vi "GetProgress.vi"(8 "error in (no error)":errorcluster, 11 "Progress in":refnum<class "Progress.lvclass">) -> (0 "error out":errorcluster, 2 "Progress":u64, 3 "Progress out":refnum<class "Progress.lvclass">)   [LabVIEW 2021, in "Progress.lvlib" / "Progress.lvclass"]
uses:
  Progress.lvclass
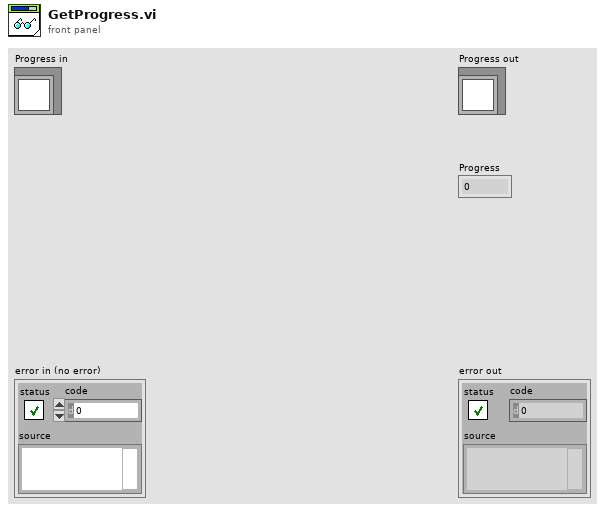
[diagram p1: front panel]
types:
  T1 = typedef "Progress.lvlib/Progress.lvclass/Data.ctl" = cluster{"SlideRefnum":refnum<vi>, "ProgressValue":u64, "NbElement":u64, "Caption":string, "UINotifier":refnum<notifier>, "StopUI":refnum<user-event>}
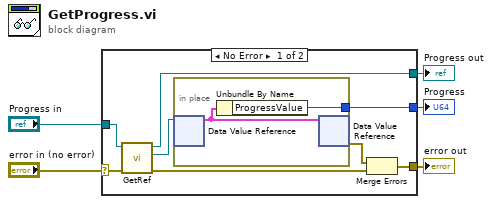
[diagram p0: block diagram]
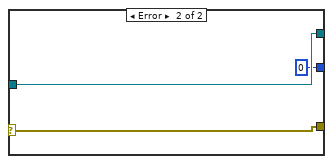
[diagram p2: hidden frame]
diagram:
  n1 = case shown="No Error" "error in (no error)" {
    selector: "error in (no error)" -> [w10 w18]
    tunnel: [w7 w18] -> w4
    tunnel: [w12 w17] -> w2
    tunnel: "Progress in" -> [w11 w17]
    tunnel: [w6 u64 0 ("ProgressValue")] -> w1
    frame No Error {
      n2 = call "GetRef.vi"("error in (no error)"=w10, "Progress in"=w11) -> ("error out"=w8:errorcluster, "ref"=w13:refnum<data-value>, "Progress out"=w12:refnum<class "Progress.lvclass">)  [unwired: 7 in]
      n3 = in-place {
        in-place-border: [w15] -> w6
        n4 = in-place-dvr #1(w13) -> (w14:T1)  [unwired: 1 out]
        n5 = Unbundle By Name(w14) -> ("ProgressValue"=w15:u64)
        n6 = in-place-dvr #1(w14) -> (w9:errorcluster)  [unwired: 1 out]
      }
      n7 = Merge Errors(w9, w8) -> (w7:errorcluster)
    }
    frame Error {
    }
  }
  "error out" <- w4
  "Progress out" <- w2
  "Progress" <- w1
